vi "Open DLL.vi"(8 "error in (no error)":errorcluster, 10 "Build specification name":string, 11 "Project Refnum":refnum<vi>) -> (0 "error out":errorcluster, 3 "DLL out":refnum<class "NI_AB_API_DLL.lvclass">)   [LabVIEW 2020, in "NI_AB_API_DLL.lvclass"]
uses:
  <vilib>/AppBuilder/AB_API/DLL/NI_AB_API_DLL.lvclass
  e:/builds/penguin/labview/branches/2020/dev/dist/vi.lib/AppBuilder/AB_API/Build/NI_AB_API_Build.lvclass
  <vilib>/AppBuilder/AB_API/common/AB_API Build Object Type.ctl
  <vilib>/AppBuilder/AB_Classes/Build/AB_Build.lvclass
  <vilib>/AppBuilder/AB_API/Build/NI_AB_API_Build.lvclass
panel:
  in  "TargetItem Refnum":refnum<vi>
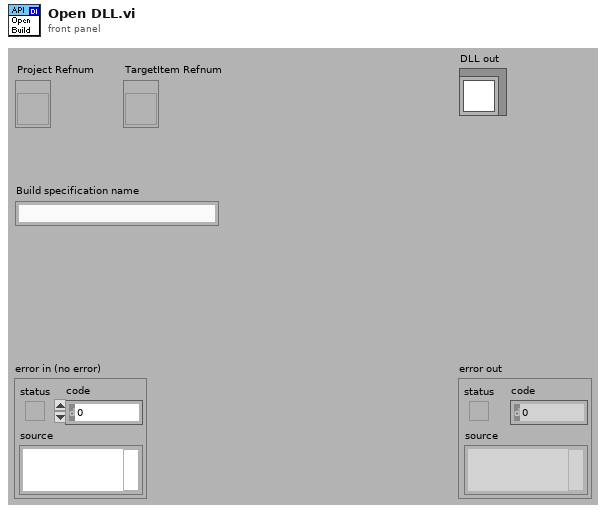
[diagram p1: front panel]
types:
  T1 = typedef "AB_API Build Object Type.ctl" = enum16{"Source Distribution", "DLL", "EXE", "Installer", "Zip File", "RESTful WS", "RTEXE", "Packed Library", "C Generation ", ".NET Interop Assembly"}
  T2 = typedef "ItemRef.ctl" = u64
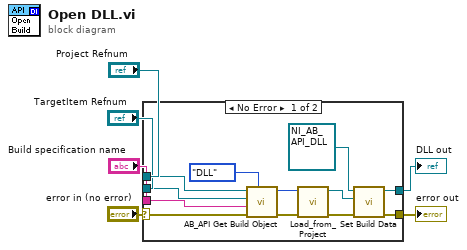
[diagram p0: block diagram]
diagram:
  n1 = case shown="No Error" "error in (no error)" {
    selector: "error in (no error)" -> [w12 w19]
    tunnel: [w10 w19] -> w5
    tunnel: [w9 _] -> w4
    tunnel: "Project Refnum" -> [w15 _]
    tunnel: "TargetItem Refnum" -> [w14 _]
    tunnel: "Build specification name" -> [w13 _]
    frame No Error {
      n2 = call <vilib>:"AB_API Get Build Object.vi"("Build object type"=AB_API_Build_Object_Type."DLL", "error in (no error)"=w12, "Build spec name"=w13, "TargetItem Refnum"=w14, "Project Refnum"=w15) -> ("error out"=w16:errorcluster, "Build Object"=w17:T2)  [unwired: 5 in]
      n3 = call <vilib>:"Load_from_Project.vi"("error in (no error)"=w16, "Object"=w17) -> ("error out"=w11:errorcluster, "Build out"=w7:refnum<class "AB_Build.lvclass">)  [unwired: 8 in]
      n4 = call <vilib>:"Set Build Data.vi"("error in (no error)"=w11, "AB_Build.lvclass"=w7, "NI_AB_API_Build in"=refnum<class "NI_AB_API_DLL.lvclass"> refnum ("NI_AB_API_DLL.lvclass")) -> ("error out"=w10:errorcluster, "NI_AB_API_Build out"=w9:refnum<class "NI_AB_API_DLL.lvclass">)  [unwired: 7 in]
    }
    frame Error {
    }
  }
  "error out" <- w5
  "DLL out" <- w4
